vi "SENS_IF_SOUR_PATH.vi"(0 "VISA IN":refnum<visa-resource-name>, 1 "ID":string, 2 "IF Input Path":string, 5 "error in":errorcluster, 7 "Channel":i32) -> (14 "VISA Out":refnum<visa-resource-name>, 19 "error out":errorcluster)   [LabVIEW 2018, in "PNA-X.lvlib"]
doc: "SENSe<cnum>:IF:SOURce:PATH <id>, <char> \n(Read Write) Sets the source path for the specified receiver. An error is returned if <id> is not valid, \nor if <char> is not valid for the specified <id>. \nParameters \n<cnum> Existing channel number to manipulate. If unspecified, <cnum> is set to 1. \n<id> Choose from: 'A', 'B', 'R1', 'R2' \nNote: The A and R1 receivers are always switched together. B and R2 are also \nalways switched together. For example, if you specify \"A\", R1 will also be \nswitched. \n<char> Choose from: \nNORMal - the PNA decides the appropriate IF input paths. \nEXTernal - always use the rear panel IF inputs. \nExamples SENS:IF:SOUR:PATH 'A', Ext \nQuery Syntax SENSe<cnum>:IF:SOURce:PATH? <id> \nReturn Type Character \nDefault Normal \n1752\n\nSense:IF Commands \nControls the IF filter for use with the PNA X. \nClick on a blue keyword to view the command details. \nSynchronizing the PNA and Controller \nSCPI Command Tree \nPNA-X DSP Block diagram \nAll of the Sense:IF commands, except the frequency commands, make settings related to the DSP section of the IF Path. \nSee the entire IF Path Configuration. \nNote: For any of the Filter \"Stage\" parameters to take effect, SENS:IF:FILT:AUTO must be set to OFF \n(MANUAL) and mode, and SENS:IF:FILT:CMOD must be set to OFF. \n1753\n\nCritical Note: These commands act on the selected measurement. You can select one measurement for \neach channel using Calc:Par:Select"
uses:
  PNA-X.lvlib
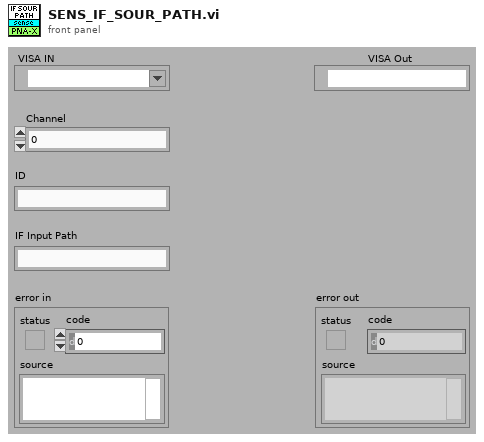
[diagram p1: front panel]
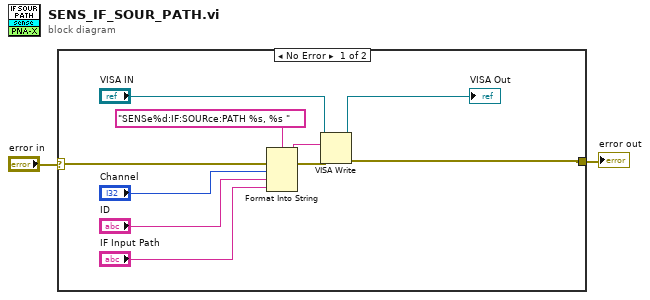
[diagram p0: block diagram]
diagram:
  n1 = case shown="No Error" "error in" {
    selector: "error in" -> [w12 w13]
    tunnel: [w7 w13] -> w1
    frame No Error {
      n2 = Format Into String(format string="SENSe%d:IF:SOURce:PATH %s, %s " ("Cmdline"), error in=w12, "Channel", "ID", "IF Input Path") -> (resulting string=w10:string, error out=w11:errorcluster)  [unwired: 1 in]
      n3 = VISA Write(VISA resource name="VISA IN", write buffer=w10, error in (no error)=w11) -> (VISA resource name out=→"VISA Out":refnum<visa-resource-name>, error out=w7:errorcluster)  [unwired: 1 out]
    }
    frame Error {
    }
  }
  "error out" <- w1
